vi "Draw.vi"(7 "3D Picture":refnum<vi>, 8 "error in (no error)":errorcluster, 11 "XRay Scene in":refnum<class "XRay Scene.lvclass">) -> (0 "error out":errorcluster, 3 "XRay Scene out":refnum<class "XRay Scene.lvclass">, 5 "Scene Object":refnum<vi>)   [LabVIEW 2026, in "XRay Scene.lvclass"]
uses:
  XRay Scene.lvclass
  XRay Scene.lvclass/XRay Scene.ctl
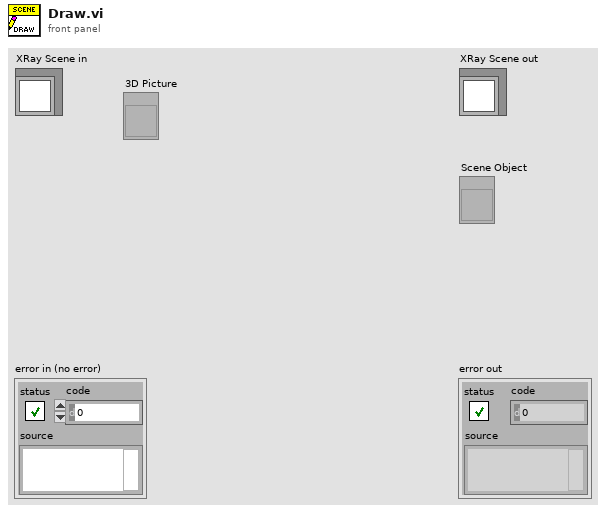
[diagram p1: front panel]
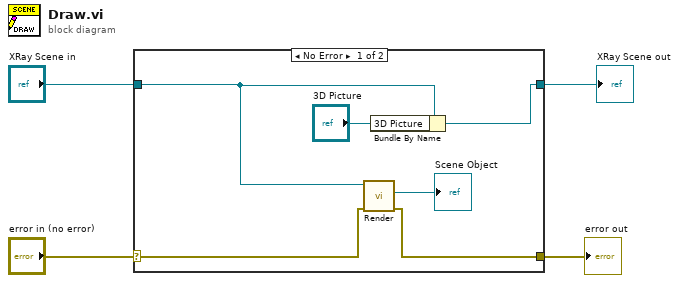
[diagram p0: block diagram]
diagram:
  n1 = case shown="No Error" "error in (no error)" {
    selector: "error in (no error)" -> [w9 w12]
    tunnel: [w8 w12] -> w3
    tunnel: "XRay Scene in" -> [w7 w11]
    tunnel: [w6 w11] -> w1
    frame No Error {
      n2 = call-dynamic "Render.vi"("error in (no error)"=w9, "XRay Scene in"=w7) -> ("error out"=w8:errorcluster, "Scene Object"=→"Scene Object":refnum<vi>)  [unwired: 7 in, 1 out]
      n3 = Bundle By Name(cluster=w7, "3D Picture"="3D Picture") -> (w6:refnum<class "XRay Scene.lvclass">)
    }
    frame Error {
    }
  }
  "error out" <- w3
  "XRay Scene out" <- w1
